vi "Example FFT.vi"() -> ()   [LabVIEW 2015]
uses:
  RTL-SDR Class/TypeDef/Device USB String.ctl
  RTL-SDR Class/RTL-SDR.lvclass
  <vilib>/Analysis/4window.llb/windowTd.ctl
  <vilib>/measure/maspectr.llb/FFT Power Spectrum and PSD for 1 Chan (CDB).vi
  <vilib>/measure/NI_MAPro.lvlib
  <vilib>/Analysis/NI_AALPro.lvlib
panel:
  in  "Center Frequency":u32=106100000
  in  "Sample Rate":u32=2400000
  out "Device USB Strings":T1
  in  "Device Index":u32
  out "Waveform Graph":cluster{"f0":dbl, "df":dbl, "magnitude":dbl[]}(graph)
  in  "stop":bool
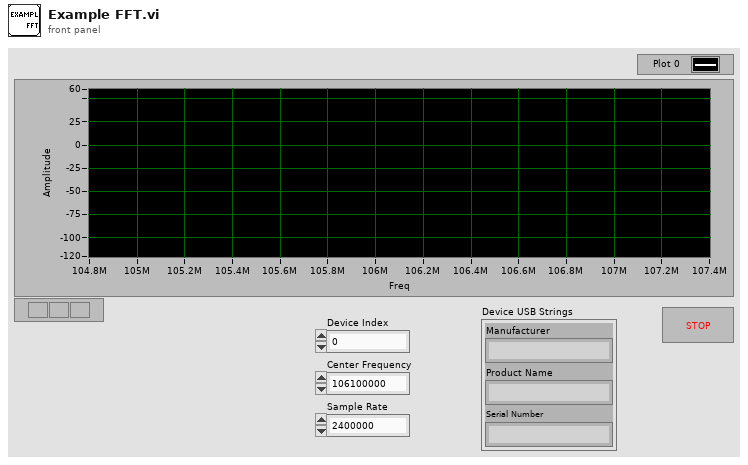
[diagram p1: front panel]
types:
  T1 = typedef "RTL-SDR.lvclass/Device USB String.ctl" = cluster{"Manufacturer":string, "Product Name":string, "Serial Number":string}
  T2 = typedef "NI_AALPro.lvlib/windowTd.ctl" = u32
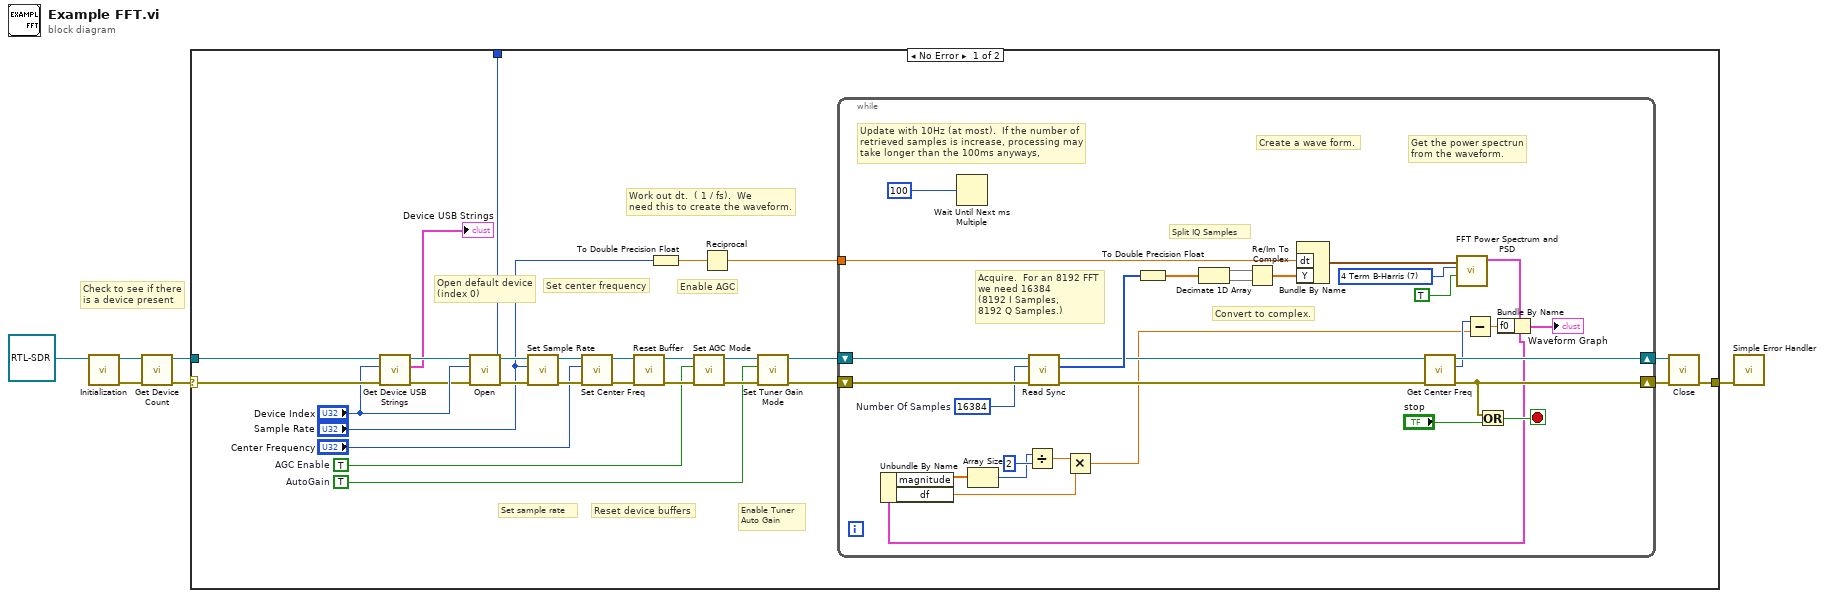
[diagram p0: block diagram]
diagram:
  # "Check to see if there\nis a device present"
  n1 = call "Initialization.vi"("RTL-SDR in"=refnum<class "RTL-SDR.lvclass"> refnum) -> ("error out"=w4:errorcluster, "RTL-SDR out"=w5:refnum<class "RTL-SDR.lvclass">)  [unwired: 8 in, 1 out]
  n2 = call "Get Device Count.vi"("error in (no error)"=w4, "RTL-SDR in"=w5) -> ("error out"=w2:errorcluster, "RTL-SDR out"=w1:refnum<class "RTL-SDR.lvclass">)  [unwired: 7 in, 1 out]
  n3 = case shown="No Error" w2 {
    selector: w2 -> [w12 w64]
    tunnel: [w14 w64] -> w6
    tunnel: w1 -> [w13 _]
    tunnel: [w7 _] -> _
    frame No Error {
      w22 = TRUE  # AutoGain
      w25 = TRUE  # AGC Enable
      # "Work out dt.  ( 1 / fs).  We\nneed this to create the waveform."
      # "Enable Tuner\nAuto Gain"
      # "Enable AGC"
      # "Reset device buffers"
      # "Set center frequency"
      # "Set sample rate"
      # "Open default device\n(index 0)"
      n4 = call "Get Device USB Strings.vi"("error in (no error)"=w12, "Device Index"="Device Index", "RTL-SDR in"=w13) -> ("error out"=w10:errorcluster, "Device USB Strings"=→"Device USB Strings":T1, "RTL-SDR out"=w9:refnum<class "RTL-SDR.lvclass">)  [unwired: 5 in, 1 out]
      n5 = call "Open.vi"("error in (no error)"=w10, "Device Index"="Device Index", "RTL-SDR in"=w9) -> ("error out"=w34:errorcluster, "function return"=w7:i32, "RTL-SDR out"=w33:refnum<class "RTL-SDR.lvclass">)  [unwired: 6 in]
      n6 = call "Set Sample Rate.vi"("error in (no error)"=w34, "Sample Rate"="Sample Rate", "RTL-SDR in"=w33) -> ("error out"=w32:errorcluster, "RTL-SDR out"=w31:refnum<class "RTL-SDR.lvclass">)  [unwired: 6 in, 1 out]
      n7 = call "Set Center Freq.vi"("error in (no error)"=w32, "Center Frequency"="Center Frequency", "RTL-SDR in"=w31) -> ("error out"=w28:errorcluster, "RTL-SDR out"=w29:refnum<class "RTL-SDR.lvclass">)  [unwired: 6 in, 1 out]
      n8 = call "Reset Buffer.vi"("error in (no error)"=w28, "RTL-SDR in"=w29) -> ("error out"=w27:errorcluster, "RTL-SDR out"=w26:refnum<class "RTL-SDR.lvclass">)  [unwired: 7 in, 1 out]
      n9 = To Double Precision Float(number="Sample Rate") -> (double precision float=w19:dbl)
      n10 = call "Set AGC Mode.vi"("error in (no error)"=w27, "AGC Enable"=w25, "RTL-SDR in"=w26) -> ("error out"=w24:errorcluster, "RTL-SDR out"=w23:refnum<class "RTL-SDR.lvclass">)  [unwired: 6 in, 1 out]
      n11 = Reciprocal(x=w19) -> (1/x=w17:dbl)
      n12 = call "Set Tuner Gain Mode.vi"("error in (no error)"=w24, "AutoGain"=w22, "RTL-SDR in"=w23) -> ("error out"=w21:errorcluster, "RTL-SDR out"=w20:refnum<class "RTL-SDR.lvclass">)  [unwired: 6 in, 1 out]
      n13 = while {
        shift-right: [w47] -> w15
        shift-left: w21 -> [w52]
        shift-right: [w46] -> w16
        shift-left: w20 -> [w51]
        tunnel: w17 -> [w42]
        stop <- w54 stop-if-true
        w45 = 16384  # Number Of Samples
        w60 = T2 7 items=["Rectangle"=0, "Hanning"=1, "Hamming"=2, "Blackman-Harris"=3, "Exact Blackman"=4, "Blackman"=5, "Flat Top"=6, "4 Term B-Harris "=7, "7 Term B-Harris"=8, "Low Sidelobe"=9, "Blackman Nuttall"=11, "Triangle"=30, "Bartlett-Hanning"=31, "Bohman"=32, "Parzen"=33, "Welch"=34, "Kaiser"=60, "Dolph-Chebyshev"=61, "Gaussian"=62] ("window")
        # "Update with 10Hz (at most).  If the number of \nretrieved samples is increase, processing may\ntake longer than the 100ms anyways,"
        # "Get the power spectrun\nfrom the waveform."
        # "Acquire.  For an 8192 FFT\nwe need 16384 \n(8192 I Samples,\n8192 Q Samples.)"
        # "Create a wave form."
        # "Convert to complex."
        # "Split IQ Samples"
        n14 = Wait Until Next ms Multiple(millisecond multiple=u32 100) -> ()  [unwired: 1 out]
        n15 = call "Read Sync.vi"("error in (no error)"=w52, "Number Of Samples"=w45, "RTL-SDR in"=w51) -> ("error out"=w48:errorcluster, "Sample Buffer"=w50:u8[], "RTL-SDR out"=w49:refnum<class "RTL-SDR.lvclass">)  [unwired: 4 in, 2 out]
        n16 = To Double Precision Float(number=w50) -> (double precision float=w63:dbl[])
        n17 = Decimate 1D Array(w63) -> (w62:dbl[], w61:dbl[])
        n18 = Re/Im To Complex(1:w61, 2:w62) -> (0:w57:cdb[])
        n19 = Bundle By Name("dt"=w42, "Y"=w57) -> (w58:waveform(cdb))  [unwired: 1 in]
        n20 = call "Get Center Freq.vi"("error in (no error)"=w48, "RTL-SDR in"=w49) -> ("error out"=w47:errorcluster, "Center Frequency"=w41:u32, "RTL-SDR out"=w46:refnum<class "RTL-SDR.lvclass">)  [unwired: 7 in]
        n21 = call-poly <vilib>:"FFT Power Spectrum and PSD.vi"("dB On (F)"=TRUE, "window"=w60, "time signal"=w58) -> ("Power Spectrum / PSD"=w38:cluster{"f0":dbl, "df":dbl, "magnitude":dbl[]})  [unwired: 5 in, 3 out]
        n22 = Unbundle By Name(w38) -> ("magnitude"=w36:dbl[], "df"=w37:dbl)
        n23 = Array Size(array=w36) -> (size(s)=w35:i32)
        n24 = Divide(x=w35, y=2) -> (x/y=w43:dbl)
        n25 = Multiply(x=w43, y=w37) -> (x*y=w40:dbl)
        n26 = Subtract(x=w41, y=w40) -> (x-y=w39:dbl)
        n27 = Or(x=w47, y="stop") -> (x .or. y?=w54:bool)
        n28 = Bundle By Name(cluster=w38, "f0"=w39) -> (→"Waveform Graph":cluster{"f0":dbl, "df":dbl, "magnitude":dbl[]})
      }
      n29 = call "Close.vi"("error in (no error)"=w15, "RTL-SDR in"=w16) -> ("error out"=w14:errorcluster)  [unwired: 7 in, 2 out]
    }
    frame Error {
    }
  }
  n30 = call <vilib>:"Simple Error Handler.vi"("error in (no error)"=w6) -> ()  [unwired: 4 in, 5 out]
